vi "Get Colors.vi"(11 "Orange Plugin in":refnum<class "Orange Plugin.lvclass">) -> (3 "Color Box":u32(colorbox))   [LabVIEW 2020, in "Orange Plugin.lvclass"]
uses:
  Orange Plugin.lvclass
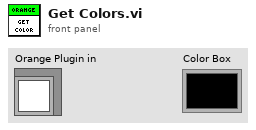
[diagram p1: front panel]
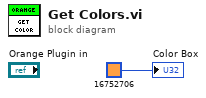
[diagram p0: block diagram]
diagram:
  "Color Box" <- u32 16752706 ("Color Box")
